vi "GetPDPCurrents.vi"(11 "Channels":i32[](array[numeric])) -> (3 "Currents":dbl[](array[numeric]))   [LabVIEW 2017]
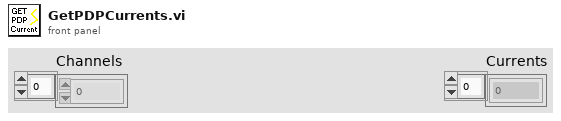
[diagram p1: front panel]
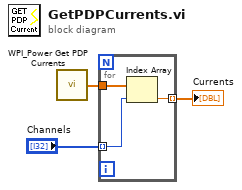
[diagram p0: block diagram]
diagram:
  n1 = call <vilib>:"WPI_Power Get PDP Currents.vi"() -> ("all currents (A)"=w3:dbl[])  [unwired: 13 in, 2 out]
  n2 = for {
    tunnel: w3 -> [w6]
    tunnel: "Channels" -> [w5] mode=indexing
    tunnel: [w4] -> w1 mode=indexing
    n3 = Index Array(array=w6, index=w5) -> (element=w4:dbl)
  }
  "Currents" <- w1
